vi "20181113_2.vi"() -> ()   [LabVIEW 2017]
panel:
  out "Waveform Chart":cluster{dbl, dbl}(graph)
  out "appended array":dbl[](array[numeric])
  in  "stop":bool
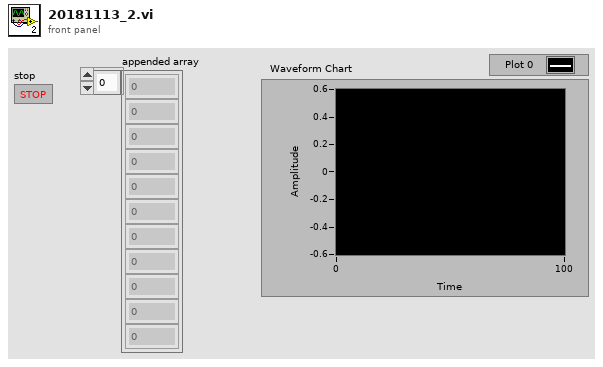
[diagram p1: front panel]
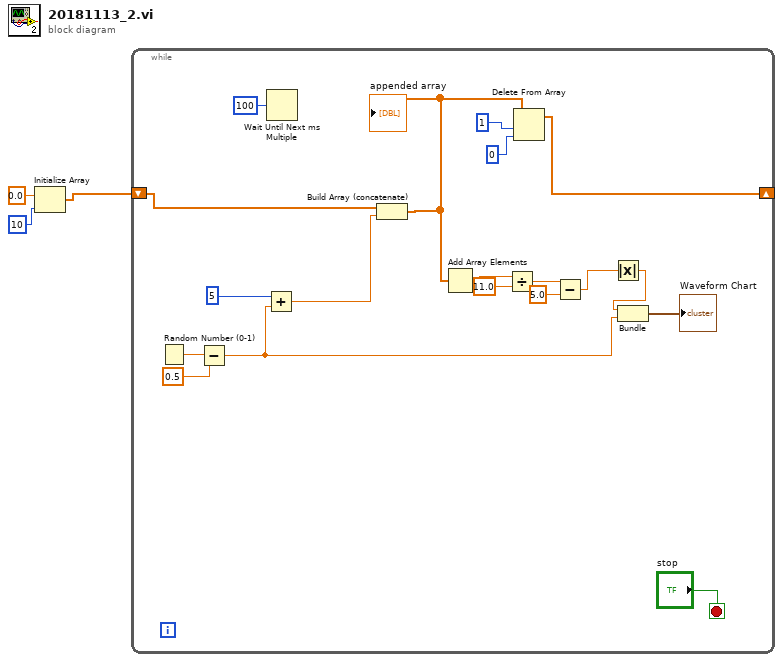
[diagram p0: block diagram]
diagram:
  n1 = Initialize Array(0.0 ("element"), 10 ("dimension size")) -> (w1:dbl[])
  n2 = while {
    shift-right: [w14] -> _
    shift-left: w1 -> [w21]
    stop <- "stop" stop-if-true
    n3 = Random Number (0-1)() -> (number: 0 to 1=w16:dbl)
    n4 = Subtract(x=w16, y=0.5) -> (x-y=w7:dbl)
    n5 = Add(x=5, y=w7) -> (x+y=w20:dbl)
    n6 = Wait Until Next ms Multiple(millisecond multiple=u32 100) -> ()  [unwired: 1 out]
    n7 = Build Array (concatenate)(w21, w20) -> (w12:dbl[])
    "appended array" <- w12
    n8 = Add Array Elements(numeric array=w12) -> (sum=w11:dbl)
    n9 = Divide(x=w11, y=11.0) -> (x/y=w9:dbl)
    n10 = Delete From Array(array=w12, length=1, index=0) -> (array with subset deleted=w14:dbl[])  [unwired: 1 out]
    n11 = Subtract(x=w9, y=5.0) -> (x-y=w5:dbl)
    n12 = Absolute Value(x=w5) -> (abs(x)=w4:dbl)
    n13 = Bundle(w4, w7) -> (→"Waveform Chart":cluster{dbl, dbl})  [unwired: 1 in]
  }
